vi "cluster2.vi"() -> ()   [LabVIEW 2021]
panel:
  out "array of clusters":T1(array[cluster])
  out "output cluster":T2
  in  "gender":bool
  in  "salary":u16
  in  "age":u8
  in  "name":string
  in  "employee":T2
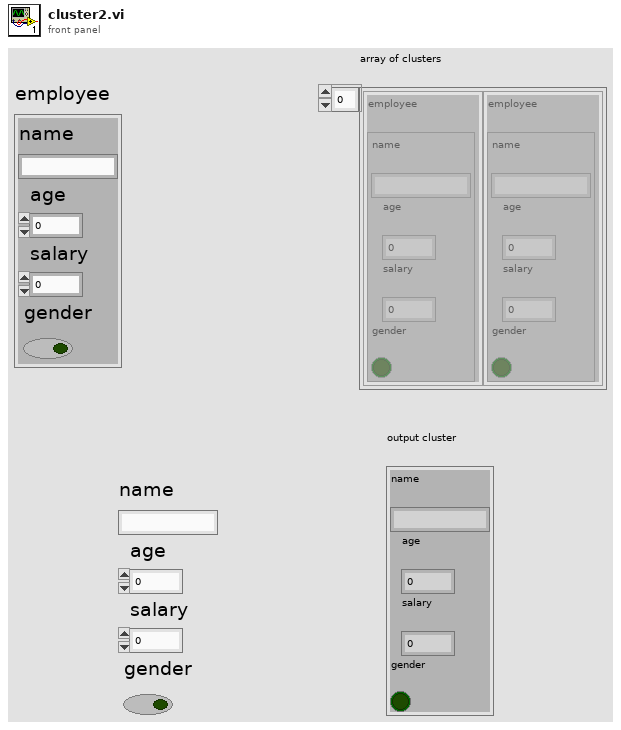
[diagram p1: front panel]
types:
  T1 = cluster{"employee":cluster{"name":string, "age":u8, "salary":u16, "gender":bool}}[]
  T2 = cluster{"name":string, "age":u8, "salary":u16, "gender":bool}
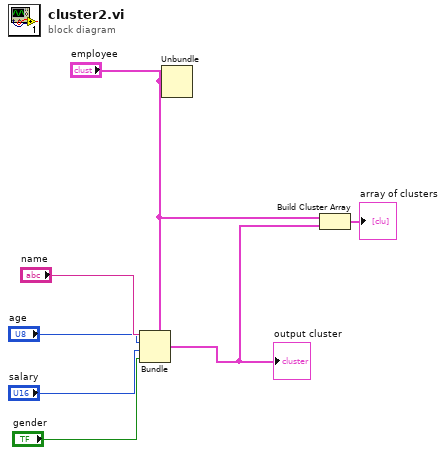
[diagram p0: block diagram]
diagram:
  n1 = Bundle(cluster="employee", "name"="name", "age"="age", "salary"="salary", "gender"="gender") -> (w2:T2)
  "output cluster" <- w2
  n2 = Unbundle("employee") -> ()  [unwired: 4 out]
  n3 = Build Cluster Array("employee", w2) -> (→"array of clusters":T1)
